vi "MTM2_issueCommand_positionMirror.vi"(8 "error in (no error)":errorcluster, 11 "command_positionMirror_Ctl":T1) -> (0 "error out":errorcluster, 2 "function return":i32, 3 "command_positionMirror_Ctl out":T1)   [LabVIEW 2018, in "SALLV_MTM2.lvlib"]
doc: "int MTM2_shm_issueCommand_positionMirrorLV(MTM2_command_positionMirrorLV *command_positionMirror_Ctl );"
uses:
  DataTypes/command_positionMirror.ctl
  SALLV_MTM2.lvlib
  SALLV_MTM2.so
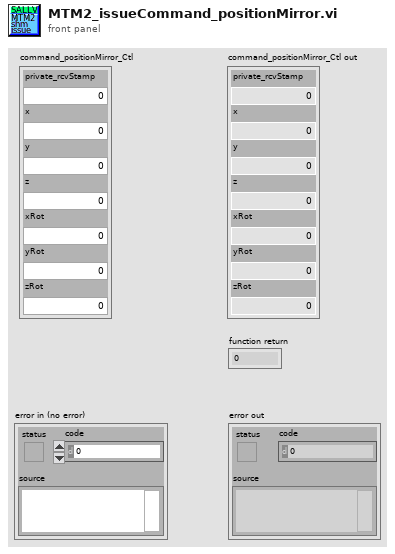
[diagram p1: front panel]
types:
  T1 = typedef "SALLV_MTM2.lvlib/command_positionMirror.ctl" = cluster{"private_rcvStamp":dbl, "x":dbl, "y":dbl, "z":dbl, "xRot":dbl, "yRot":dbl, "zRot":dbl}
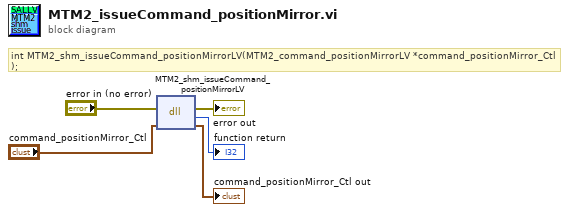
[diagram p0: block diagram]
diagram:
  # "int MTM2_shm_issueCommand_positionMirrorLV(MTM2_command_positionMirrorLV *command_positionMirror_Ctl );"
  n1 = dll-call lib="home/ttsai/Documents/salLabviewApi/SALLV_MTM2/SALLV_MTM2.*" fn="MTM2_shm_issueCommand_positionMirrorLV"(error in="error in (no error)", "command_positionMirror_Ctl"="command_positionMirror_Ctl") -> (error out=→"error out":errorcluster, →"function return":i32, "command_positionMirror_Ctl"=→"command_positionMirror_Ctl out":T1)  [unwired: 2 in, 1 out]
